vi "Determine Warning Bad One.vi"(6 "최대 풍속":dbl, 7 "현재 풍속":dbl, 8 "에러 입력(에러 없음)":errorcluster, 9 "최저 온도":dbl, 10 "최대 온도":dbl caption="최고 온도", 11 "현재 온도":dbl) -> (0 "에러 출력":errorcluster, 1 "경고?":bool caption="정지", 2 "경고 텍스트":string caption="텍스트")   [LabVIEW 2018]
doc: "이 VI는 LabVIEW Basics II에서 사용되는 연습문제 VI입니다. 향상시켜야 할 상속된 코드이 예제입니다. VI의 기능을 변경하지 않고 읽기와 관리가 보다 쉽도록 개선하십시오."
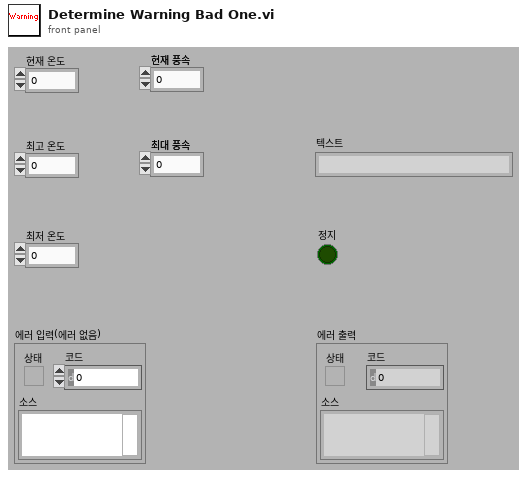
[diagram p1: front panel]
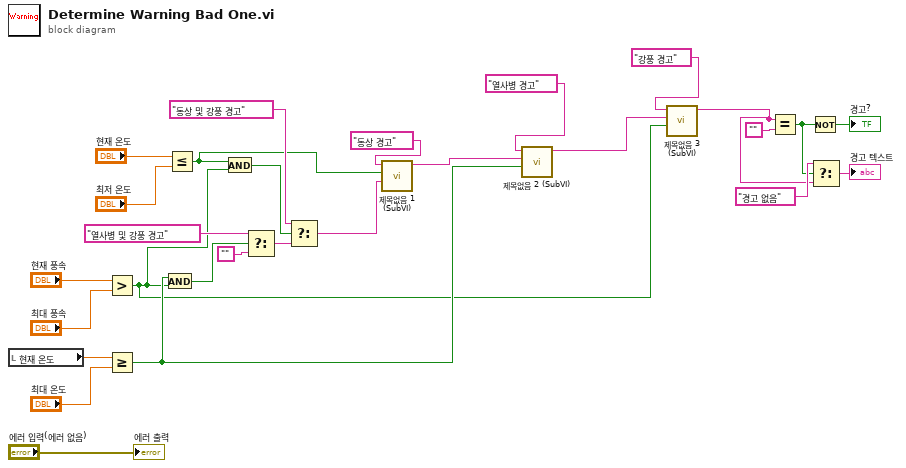
[diagram p0: block diagram]
diagram:
  n1 = local read "현재 온도"() -> (w4:dbl)
  n2 = Greater?(x="현재 풍속", y="최대 풍속") -> (0:w13:bool)
  n3 = Greater Or Equal?(x=w4, y="최대 온도") -> (x >= y?=w14:bool)
  n4 = And(x=w14, y=w13) -> (x .and. y?=w21:bool)
  n5 = Less Or Equal?(x="현재 온도", y="최저 온도") -> (x <= y?=w17:bool)
  n6 = And(x=w17, y=w13) -> (x .and. y?=w18:bool)
  n7 = Select(t="열사병 및 강풍 경고", s=w21, f="") -> (s? t:f=w10:string)
  n8 = Select(t="동상 및 강풍 경고", s=w18, f=w10) -> (s? t:f=w9:string)
  n9 = call "제목없음 1 (SubVI).vi"("문자열 입력"=w9, "불리언"=w17, "문자열 3"="동상 경고") -> ("문자열 출력"=w7:string)  [unwired: 8 in]
  n10 = call "제목없음 2 (SubVI).vi"("불리언"=w14, "문자열 입력"=w7, "문자열"="열사병 경고") -> ("문자열 출력 2"=w8:string)  [unwired: 8 in]
  n11 = call "제목없음 3 (SubVI).vi"("불리언"=w13, "문자열 출력 3"=w8, "문자열"="강풍 경고") -> ("문자열 출력 2"=w5:string)  [unwired: 8 in]
  n12 = Equal?(x=w5, y="") -> (x = y?=w2:bool)
  n13 = Not(x=w2) -> (.not. x?=→"경고?":bool)
  n14 = Select(t="경고 없음" ("f"), s=w2, f=w5) -> (s? t:f=→"경고 텍스트":string)
  "에러 출력" <- "에러 입력(에러 없음)"
